vi "Select XNET Signals.vi"(8 "error in (no error)":errorcluster, 11 "Node Ptr":u64 format="%.0x") -> (0 "error out":errorcluster)   [LabVIEW 2025, in "Protection and Counter Addon System Explorer.lvlib"]
uses:
  Protection and Counter Addon System Explorer.lvlib
  Addon Shared/SubVIs/GUID Lookup.vi
  Addon Shared/Protection and Counter Addon Shared.lvlib
panel:
  in  "Tag":string
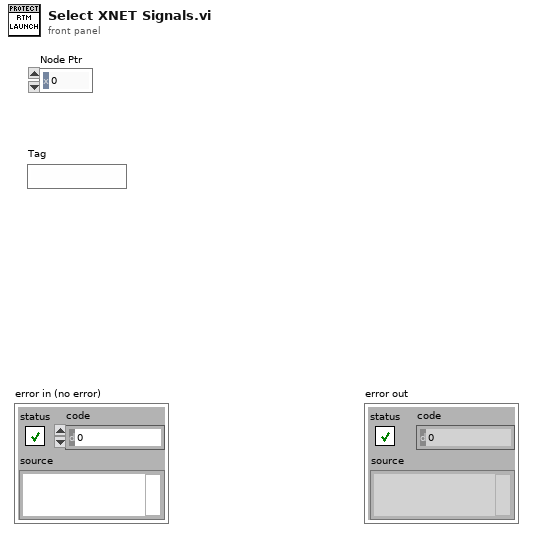
[diagram p1: front panel]
types:
  T1 = typedef "Custom Device API.lvlib/Custom Device Item Ref.ctl" = u64
  T2 = typedef "Protection and Counter Addon Shared.lvlib/XNET Settings.ctl" = cluster{"Database":refnum<k21>, "Cluster":refnum<k21>, "Port":string, "Baud rate [Bd]":u64, "Termination":u32, "CAN I/O Mode":u32, "FD Baud rate [Bd]":u64, "Priority":i32, "Use Legacy":bool, "FD ISO Mode":u32, "Default Max Counter Value":dbl, "Default Protect Type":T3}
  T3 = typedef "Protection and Counter Support Shared.lvlib/Protection Type.ctl" = enum16{"Arb ID + Bytes Checksum with Inversion", "Arb ID + Bytes CRC with Inversion", "Reversed Raw Signal Checksum with Inversion", "Concatenated Two's Compliment"}
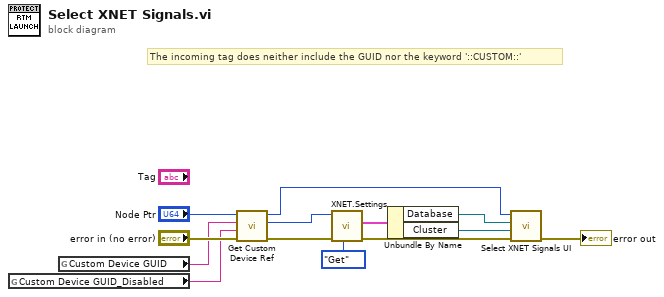
[diagram p0: block diagram]
diagram:
  # "The incoming tag does neither include the GUID nor the keyword '::CUSTOM::'"
  n1 = global read "GUID Lookup.vi" "Custom Device GUID_Disabled"() -> (w1:string)
  n2 = global read "GUID Lookup.vi" "Custom Device GUID"() -> (w2:string)
  n3 = call "Get Custom Device Ref.vi"("error in"="error in (no error)", "Custom Device GUID_Disabled"=w1, "Custom Device GUID"=w2, "Section Ptr"="Node Ptr") -> ("error out"=w9:errorcluster, "Custom Device Ref"=w10:T1, "Section Ref out"=w11:T1)  [unwired: 5 in]
  n4 = call "XNET.Settings.vi"("Action"=enum8{"Get", "Set"}."Get", "error in (no error)"=w9, "Parent Ref in"=w10) -> ("error out"=w8:errorcluster, "XNET Settings"=w5:T2)  [unwired: 6 in, 1 out]
  n5 = Unbundle By Name(w5) -> ("Database"=w7:refnum<k21>, "Cluster"=w6:refnum<k21>)
  n6 = call "Select XNET Signals UI.vi"("error in (no error)"=w8, "XNET Cluster"=w6, "XNET Database"=w7, "Node Ptr"=w11) -> ("error out"=→"error out":errorcluster)  [unwired: 5 in, 2 out]
